vi "VI_Heat_Tape_Final_duplicate.vi"() -> ()   [LabVIEW 2019]
uses:
  <vilib>/NI/Modbus Library/API/Wrapper/Create Serial Master.vi
  <vilib>/NI/Modbus Library/API/Master/Modbus Master.lvclass
  <vilib>/NI/Modbus Library/API/Wrapper/API Main.lvlib
  <vilib>/NI/Modbus Library/Transmission Data Unit/RTU/RTU Data Unit.lvclass
panel:
  out "Value 4":sgl
  out "Value 3":sgl
  out "Connection Status":bool
  in  "unit ID (Defaut: 1)":u8=1
  in  "number of inputs (Defaut: 60)":u16
  in  "starting address (Default: 1)":u16
  in  "Flow Control (Default: None)":u16(ring) items=["None", "XON/XOFF", "RTS/CTS", "XON/XOFF & RTS/CTS", "DTR/DSR", "XON/XOFF & DTR/DSR"]
  in  "Serial Type (Default: RTU)":enum16{"RTU", "ASCII"}(ring)
  in  "Parity (Default: None)":u16(ring)=2 items=["None", "Odd", "Even", "Mark", "Space"]
  in  "Baud Rate (Default: 115400)":u32=9600
  in  "COM Port (Default: COM7)":refnum<visa-resource-name>
  in  "Set Value":string
  out "Alarm Status":bool
  out "?":cluster{dbl, dbl}(graph)
  out "Heater Status":bool
  in  "Hysterisis Value":string
  out "Current Temperature Status":bool
  in  "?":bool
  out "Current Temperature (ºF)":string
  out "Heat Tape 01  Temperature (ºF)":dbl(slide) scale=65.0..85.0
  out "Query Message":string
  out "Register and RAW value":u16[](array[numeric])
  in  "error check":errorcluster
  # "SpinQuest Heat Tape Temperature Monitoring System"
  # "PXF4 Settings"
  # "RS-485 Connection"
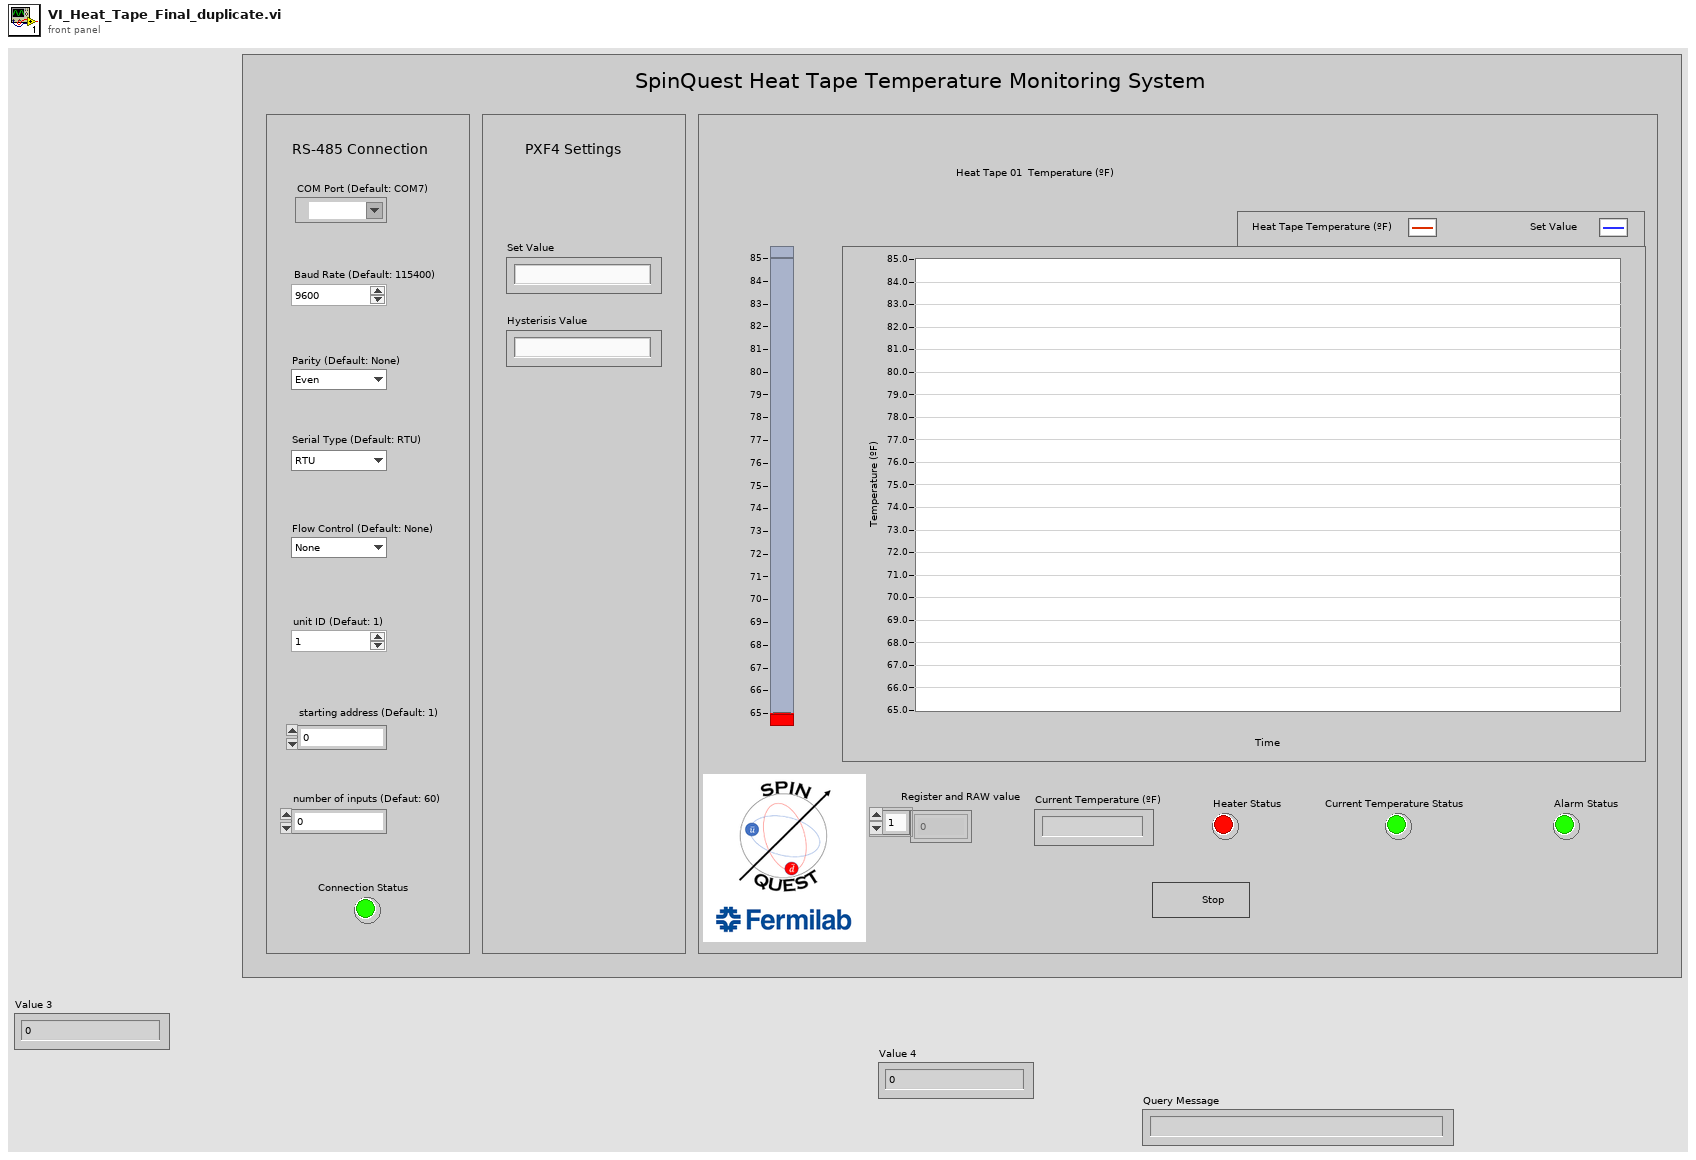
[diagram p1: front panel]
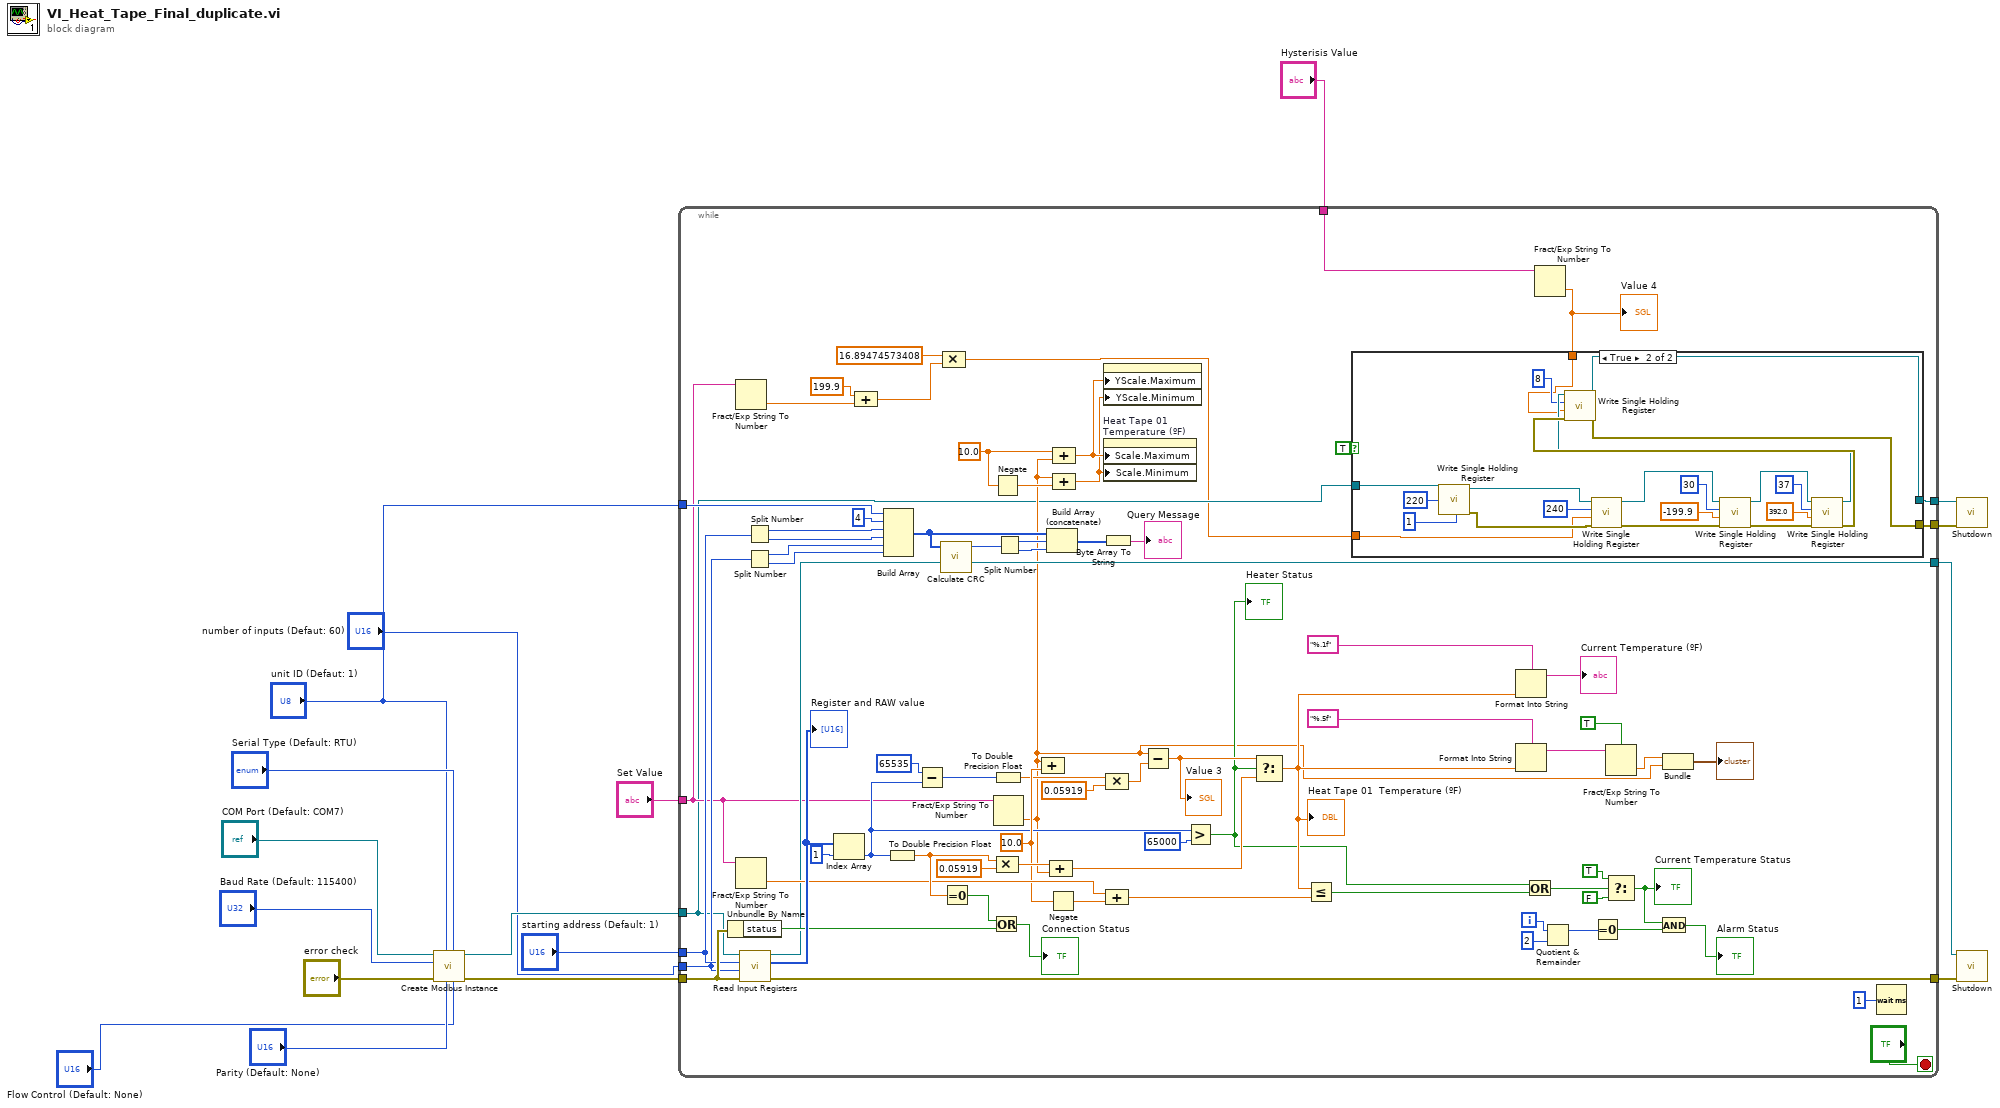
[diagram p0: block diagram]
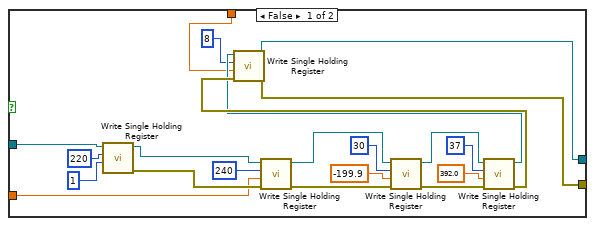
[diagram p2: hidden frame]
diagram:
  n1 = call-poly <vilib>:"Create Modbus Instance.vi"("flow control (none)"="Flow Control (Default: None)", "serial type"="Serial Type (Default: RTU)", "parity (even)"="Parity (Default: None)", "unit ID"="unit ID (Defaut: 1)", "error in"="error check", "baud rate"="Baud Rate (Default: 115400)", "VISA resource name"="COM Port (Default: COM7)") -> ("error out"=w11:errorcluster, "serial master instance"=w12:refnum<class "Modbus Master.lvclass">)  [unwired: 3 in]
  n2 = while {
    tunnel: w12 -> [w19]
    tunnel: w11 -> [w59]
    tunnel: [w60] -> w9
    tunnel: [w49] -> w7
    tunnel: "unit ID (Defaut: 1)" -> [w93]
    tunnel: [w23] -> w6
    tunnel: [w24] -> w5
    tunnel: "starting address (Default: 1)" -> [w27]
    tunnel: "number of inputs (Defaut: 60)" -> [w26]
    tunnel: "Set Value" -> [w25]
    tunnel: "Hysterisis Value" -> [w21]
    i -> [w64]
    stop <- "?" stop-if-true
    w41 = 10.0 ("value")
    w51 = 10.0 ("value")
    n3 = Unbundle By Name(w59) -> ("status"=w56:bool)
    n4 = Fract/Exp String To Number(string=w25) -> (number=w48:dbl)  [unwired: 3 in, 1 out]
    n5 = Fract/Exp String To Number(string=w25) -> (number=w52:dbl)  [unwired: 3 in, 1 out]
    n6 = call-dynamic "Read Input Registers.vi"("error in"=w59, "number of inputs"=w26, "starting address"=w27, "Modbus master in"=w19) -> ("error out"=w60:errorcluster, "register values"=w79:u16[], "Modbus master out"=w49:refnum<class "Modbus Master.lvclass">)  [unwired: 5 in]
    "Register and RAW value" <- w79
    n7 = Split Number(x=w27) -> (hi(x)=w85:u8, lo(x)=w84:u8)
    n8 = Split Number(x=w26) -> (hi(x)=w83:u8, lo(x)=w82:u8)
    n9 = Index Array(array=w79, index=1) -> (element=w42:u16)
    n10 = Compound Arithmetic op=unknown(199.9 ("value"), w48) -> (w46:dbl)
    n11 = Build Array(w93, u8 4 ("element"), w85, w84, w83, w82) -> (w91:u8[])
    n12 = To Double Precision Float(number=w42) -> (double precision float=w58:dbl)
    n13 = Subtract(x=u16 65535 ("y"), y=w42) -> (x-y=w33:u16)
    n14 = call <vilib>:"Calculate CRC.vi"("data"=w91) -> ("CRC-16"=w90:u16)  [unwired: 10 in]
    n15 = Equal To 0?(x=w58) -> (x = 0?=w55:bool)
    n16 = Compound Arithmetic op=MULTIPLY(16.89474573408 ("value"), w46) -> (w18:dbl)
    n17 = Or(x=w55, y=w56) -> (x .or. y?=→"Connection Status":bool)
    n18 = Negate(x=w41) -> (-x=w40:dbl)
    n19 = To Double Precision Float(number=w33) -> (double precision float=w35:dbl)
    n20 = Fract/Exp String To Number(string=w25) -> (number=w28:dbl)  [unwired: 3 in, 1 out]
    n21 = Split Number(x=w90) -> (hi(x)=w89:u8, lo(x)=w88:u8)
    n22 = Compound Arithmetic op=MULTIPLY(w58, 0.05919 ("value")) -> (w77:dbl)
    n23 = Compound Arithmetic op=unknown(w28, w51) -> ()  [unwired: 1 out]
    n24 = Build Array (concatenate)(w91, w89, w88) -> (w87:u8[])
    n25 = Negate(x=w51) -> (-x=w50:dbl)
    n26 = Compound Arithmetic op=ADD(w77, w28) -> (w30:dbl)
    n27 = Compound Arithmetic op=unknown(w41, w28) -> (w39:dbl)
    n28 = Compound Arithmetic op=unknown(w28, w40) -> (w38:dbl)
    n29 = Byte Array To String(unsigned byte array=w87) -> (string=→"Query Message":string)
    n30 = property class="WFChart (strict)"("YScale.Maximum"=w39, "YScale.Minimum"=w38) -> ()  [unwired: 2 in, 2 out]
    n31 = property on="Heat Tape 01  Temperature (ºF)" class="Slide (strict)"("Scale.Maximum"=w39, "Scale.Minimum"=w38) -> ()  [unwired: 2 in, 2 out]
    n32 = Compound Arithmetic op=MULTIPLY(w35, 0.05919 ("value")) -> (w32:dbl)
    n33 = Compound Arithmetic op=unknown(w52, w50) -> (w37:dbl)
    n34 = Subtract(x=w28, y=w32) -> (x-y=w31:dbl)
    "Value 3" <- w31
    n35 = Greater?(x=w42, y=u16 65000) -> (0:w29:bool)
    "Heater Status" <- w29
    n36 = Select(t=w31, s=w29, f=w30) -> (s? t:f=w36:dbl)
    "Heat Tape 01  Temperature (ºF)" <- w36
    n37 = Less Or Equal?(x=w36, y=w37) -> (x <= y?=w70:bool)
    n38 = Format Into String(format string="%.1f", w36) -> (resulting string=→"Current Temperature (ºF)":string)  [unwired: 2 in, 1 out]
    n39 = Format Into String(format string="%.5f", w36) -> (resulting string=w72:string)  [unwired: 2 in, 1 out]
    n40 = Or(x=w29, y=w70) -> (x .or. y?=w69:bool)
    n41 = Fract/Exp String To Number(string=w21) -> (number=w22:dbl)  [unwired: 3 in, 1 out]
    "Value 4" <- w22
    n42 = case shown="True" TRUE {
      tunnel: [w102 w125] -> w24
      tunnel: [w101 w123] -> w23
      tunnel: w22 -> [w100 w121]
      tunnel: w19 -> [w97 w118]
      tunnel: w18 -> [w94 w115]
      frame False {
        n43 = call-dynamic "Write Single Holding Register.vi"("register to write"=u16 1, "address"=u16 220, "Modbus master in"=w97) -> ("error out"=w95:errorcluster, "Modbus master out"=w96:refnum<class "Modbus Master.lvclass">)  [unwired: 7 in]
        n44 = call-dynamic "Write Single Holding Register.vi"("error in"=w95, "register to write"=w94, "address"=u16 240, "Modbus master in"=w96) -> ("error out"=w112:errorcluster, "Modbus master out"=w111:refnum<class "Modbus Master.lvclass">)  [unwired: 6 in]
        n45 = call-dynamic "Write Single Holding Register.vi"("error in"=w112, "register to write"=-199.9 ("value"), "address"=u16 30, "Modbus master in"=w111) -> ("error out"=w113:errorcluster, "Modbus master out"=w114:refnum<class "Modbus Master.lvclass">)  [unwired: 6 in]
        n46 = call-dynamic "Write Single Holding Register.vi"("error in"=w113, "register to write"=392.0 ("value"), "address"=u16 37, "Modbus master in"=w114) -> ("error out"=w105:errorcluster, "Modbus master out"=w104:refnum<class "Modbus Master.lvclass">)  [unwired: 6 in]
        n47 = call-dynamic "Write Single Holding Register.vi"("error in"=w105, "register to write"=w100, "address"=u16 8, "Modbus master in"=w104) -> ("error out"=w102:errorcluster, "Modbus master out"=w101:refnum<class "Modbus Master.lvclass">)  [unwired: 6 in]
      }
      frame True {
        n48 = call-dynamic "Write Single Holding Register.vi"("register to write"=u16 1, "address"=u16 220, "Modbus master in"=w118) -> ("error out"=w116:errorcluster, "Modbus master out"=w117:refnum<class "Modbus Master.lvclass">)  [unwired: 7 in]
        n49 = call-dynamic "Write Single Holding Register.vi"("error in"=w116, "register to write"=w115, "address"=u16 240, "Modbus master in"=w117) -> ("error out"=w133:errorcluster, "Modbus master out"=w132:refnum<class "Modbus Master.lvclass">)  [unwired: 6 in]
        n50 = call-dynamic "Write Single Holding Register.vi"("error in"=w133, "register to write"=-199.9 ("value"), "address"=u16 30, "Modbus master in"=w132) -> ("error out"=w134:errorcluster, "Modbus master out"=w135:refnum<class "Modbus Master.lvclass">)  [unwired: 6 in]
        n51 = call-dynamic "Write Single Holding Register.vi"("error in"=w134, "register to write"=392.0 ("value"), "address"=u16 37, "Modbus master in"=w135) -> ("error out"=w126:errorcluster, "Modbus master out"=w124:refnum<class "Modbus Master.lvclass">)  [unwired: 6 in]
        n52 = call-dynamic "Write Single Holding Register.vi"("error in"=w126, "register to write"=w121, "address"=u16 8, "Modbus master in"=w124) -> ("error out"=w125:errorcluster, "Modbus master out"=w123:refnum<class "Modbus Master.lvclass">)  [unwired: 6 in]
      }
    }
    n53 = Quotient & Remainder(x=w64, y=2) -> (x-y*floor(x/y)=w66:i32)  [unwired: 1 out]
    n54 = Equal To 0?(x=w66) -> (x = 0?=w63:bool)
    n55 = Fract/Exp String To Number(use system decimal point (T)=TRUE, string=w72) -> (number=w54:dbl)  [unwired: 2 in, 1 out]
    n56 = Select(t=TRUE, s=w69, f=FALSE) -> (s? t:f=w62:bool)
    "Current Temperature Status" <- w62
    n57 = And(x=w62, y=w63) -> (x .and. y?=→"Alarm Status":bool)
    n58 = Bundle(w54, w28) -> (→"?":cluster{dbl, dbl})  [unwired: 1 in]
    n59 = Wait (ms)(milliseconds to wait=u32 1) -> ()  [unwired: 1 out]
  }
  n60 = call-dynamic "Shutdown.vi"("error in"=w5, "Modbus master in"=w6) -> ()  [unwired: 9 in, 1 out]
  n61 = call-dynamic "Shutdown.vi"("error in"=w9, "Modbus master in"=w7) -> ()  [unwired: 9 in, 1 out]
